vi "getMovement.vi"(8 "robotPosition":T2, 10 "targetAngle":dbl=90.0 format="%#_13g", 11 "pathSegment":T1={"Point 1"={"X"=0.0, "Y"=0.0}, "Point 2"={"X"=0.0, "Y"=4000.0}}) -> (0 "finshed":bool, 1 "Rotational Velocity":dbl, 2 "Left":dbl, 3 "Forwards":dbl)   [LabVIEW 2015]
uses:
  <vilib>/vision/NI_Vision_Development_Module.lvlib
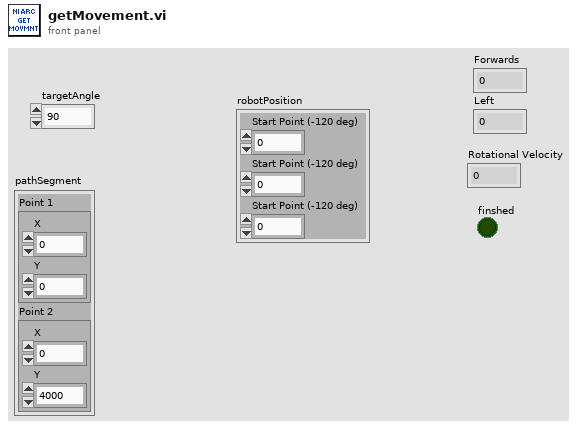
[diagram p1: front panel]
types:
  T1 = cluster{"Point 1":cluster{"X":sgl, "Y":sgl}, "Point 2":cluster{"X":sgl, "Y":sgl}}
  T2 = cluster{"Start Point (-120 deg)":dbl, "Start Point (-120 deg)":dbl, "Start Point (-120 deg)":dbl}
  T3 = cluster{"Start Point (-120 deg)":dbl, "Start Point (-120 deg)":dbl}
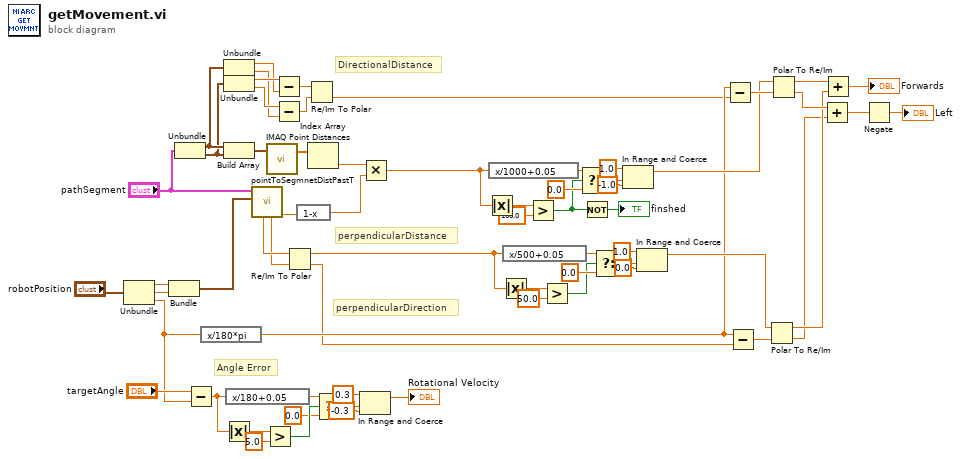
[diagram p0: block diagram]
diagram:
  # "perpendicularDirection"
  # "perpendicularDistance"
  # "DirectionalDistance"
  # "Angle Error"
  n1 = Unbundle("robotPosition") -> ("Start Point (-120 deg)"=w53:dbl, "Start Point (-120 deg)"=w52:dbl, "Start Point (-120 deg)"=w6:dbl)
  n2 = Bundle("Start Point (-120 deg)"=w53, "Start Point (-120 deg)"=w52) -> (w51:T3)  [unwired: 1 in]
  n3 = Unbundle("pathSegment") -> ("Point 1"=w25:cluster{"X":sgl, "Y":sgl}, "Point 2"=w24:cluster{"X":sgl, "Y":sgl})
  n4 = Subtract(x="targetAngle", y=w6) -> (x-y=w62:dbl)
  n5 = expression code="x/180*pi"(w6) -> (w5:dbl)
  n6 = Unbundle(w25) -> ("X"=w22:sgl, "Y"=w20:sgl)
  n7 = Unbundle(w24) -> ("X"=w23:sgl, "Y"=w21:sgl)
  n8 = Build Array(w25, w24) -> (w47:cluster{"X":sgl, "Y":sgl}[])
  n9 = Absolute Value(x=w62) -> (abs(x)=w61:dbl)
  n10 = expression code="x/180+0.05"(w62) -> (w63:dbl)
  n11 = call "pointToSegmnetDistPastT.vi"("point"=w51, "Line Segment"="pathSegment") -> ("t"=w8:dbl, "y-dist"=w49:dbl, "x-Dist"=w50:dbl)  [unwired: 5 in, 2 out]
  n12 = Greater?(x=w61, y=5.0) -> (0:w59:bool)
  n13 = call "IMAQ Point Distances"("Points"=w47) -> ("Distances"=w46:sgl[])  [unwired: 4 in, 1 out]
  n14 = Subtract(x=w23, y=w22) -> (x-y=w19:sgl)
  n15 = Subtract(x=w21, y=w20) -> (x-y=w18:sgl)
  n16 = Re/Im To Polar(2:w49, 3:w50) -> (0:w4:dbl, 1:w36:dbl)
  n17 = expression code="1-x"(w8) -> (w7:dbl)
  n18 = Re/Im To Polar(2:w18, 3:w19) -> (0:w3:sgl)  [unwired: 1 out]
  n19 = Index Array(array=w46) -> (element=w45:sgl)  [unwired: 1 in]
  n20 = Select(t=w63, s=w59, f=0.0) -> (s? t:f=w57:dbl)
  n21 = In Range and Coerce(upper limit=0.3, x=w57, lower limit=-0.3) -> (coerced(x)=→"Rotational Velocity":dbl)  [unwired: 1 out]
  n22 = Multiply(x=w45, y=w7) -> (x*y=w28:dbl)
  n23 = Absolute Value(x=w28) -> (abs(x)=w34:dbl)
  n24 = expression code="x/1000+0.05"(w28) -> (w35:dbl)
  n25 = Absolute Value(x=w36) -> (abs(x)=w38:dbl)
  n26 = expression code="x/500+0.05"(w36) -> (w37:dbl)
  n27 = Greater?(x=w34, y=100.0) -> (0:w27:bool)
  n28 = Greater?(x=w38, y=50.0) -> (0:w40:bool)
  n29 = Select(t=w35, s=w27, f=0.0) -> (s? t:f=w31:dbl)
  n30 = Not(x=w27) -> (.not. x?=→"finshed":bool)
  n31 = Select(t=w37, s=w40, f=0.0) -> (s? t:f=w42:dbl)
  n32 = In Range and Coerce(upper limit=1.0, x=w31, lower limit=-1.0) -> (coerced(x)=w14:dbl)  [unwired: 1 out]
  n33 = In Range and Coerce(upper limit=1.0, x=w42, lower limit=0.0) -> (coerced(x)=w16:dbl)  [unwired: 1 out]
  n34 = Subtract(x=w5, y=w3) -> (x-y=w15:dbl)
  n35 = Subtract(x=w5, y=w4) -> (x-y=w17:dbl)
  n36 = Polar To Re/Im(2:w17, 3:w16) -> (0:w10:dbl, 1:w11:dbl)
  n37 = Polar To Re/Im(2:w15, 3:w14) -> (0:w12:dbl, 1:w13:dbl)
  n38 = Add(x=w12, y=w10) -> (x+y=w2:dbl)
  n39 = Add(x=w13, y=w11) -> (x+y=→"Forwards":dbl)
  n40 = Negate(x=w2) -> (-x=→"Left":dbl)
